vi "Check Type.vi"(11 "Buffer Configuration":T1) -> (3 "Type":T2)   [LabVIEW 2021, in "CIF_CIPC_Chn.lvclass"]
uses:
  <vilib>/Utility/Data Type/Type Definitions/Data Type.ctl
  <vilib>/Utility/error.llb/Trim Whitespace.vi
  CIF_CIPC_Chn.lvclass
  CIF_CIPC_Chn.lvclass/CIF_CIPC_Chn.ctl
  <vilib>/CIF Foundation/CIF CIPC/CIF_NI_CIPC.lvlib
  <vilib>/Utility/Data Type/NI_Data Type.lvlib
  Typedef/Buffer Configuration Data.ctl
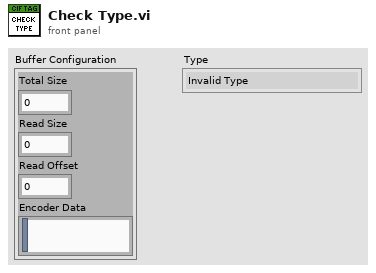
[diagram p1: front panel]
types:
  T1 = typedef "CIF_CIPC_Chn.lvclass/Buffer Configuration Data.ctl" = cluster{"Total Size":u32, "Read Size":u32, "Read Offset":u32, "Encoder Data":string}
  T2 = typedef "NI_Data Type.lvlib/Data Type.ctl" = enum8{"Invalid Type", "Void", "I8", "I16", "I32", "I64", "U8", "U16", "U32", "U64", "Single Float", "Double Float", "Extended Float", "Single Complex", "Double Complex", "Extended Complex", "Enum U8", "Enum U16", "Enum U32", "Enum U64", "Single Float With Unit", "Double Float With Unit", "Extended Float With Unit", "Single Complex with Unit", "Double Complex with Unit", "Extended Complex with Unit", "Boolean", "String", "Path", "Picture", "Tag", "Array", "Cluster", "Variant", "LV Variant", "Waveform", "Timestamp", "Digital Waveform", "Digital Data", "ExpressData", "Refnum", "External Data", "VI", "Poly VI", "LabVIEW Class Instance", "Fixed Point", "Set Collection", "Map Collection"}
  T3 = typedef "CIF_NI_CIPC.lvlib/Data Element.ctl" = cluster{"Name":string, "Type":T2, "Size":u32, "Offset":u32}
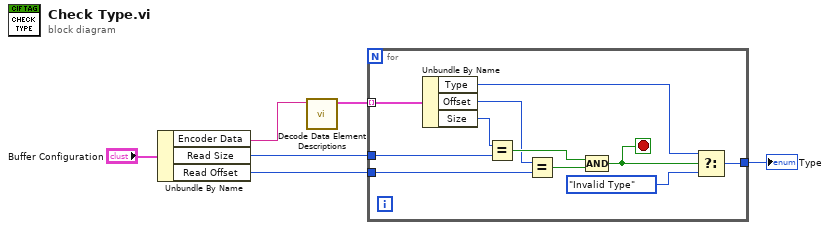
[diagram p0: block diagram]
diagram:
  n1 = Unbundle By Name("Buffer Configuration") -> ("Encoder Data"=w2:string, "Read Size"=w3:u32, "Read Offset"=w4:u32)
  n2 = call <vilib>:"Decode Data Element Descriptions.vi"("Encoder Data Description"=w2) -> ("Data Elements"=w6:T3[])  [unwired: 10 in]
  n3 = for {
    tunnel: w6 -> [w16] mode=indexing
    tunnel: w4 -> [w15]
    tunnel: w3 -> [w14]
    tunnel: [w8] -> w1
    stop <- w7 stop-if-true
    n4 = Unbundle By Name(w16) -> ("Type"=w9:T2, "Offset"=w10:u32, "Size"=w13:u32)
    n5 = Equal?(x=w13, y=w14) -> (x = y?=w12:bool)
    n6 = Equal?(x=w10, y=w15) -> (x = y?=w11:bool)
    n7 = Compound Arithmetic op=AND(w12, w11) -> (w7:bool)
    n8 = Select(t=w9, s=w7, f=Data_Type."Invalid Type") -> (s? t:f=w8:T2)
  }
  "Type" <- w1
